vi "Run.vi"(7 "Tester":refnum<class "Tester.lvclass">, 8 "error in (no error)":errorcluster, 11 "Step in":refnum<class "Step.lvclass">) -> (0 "error out":errorcluster, 3 "Step out":refnum<class "Step.lvclass">)   [LabVIEW 2020, in "Tester.lvlib" / "Step.lvclass"]
uses:
  Step.lvclass
  Tester/Tester.lvclass
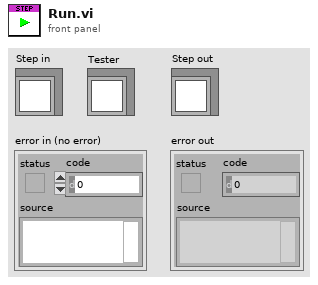
[diagram p1: front panel]
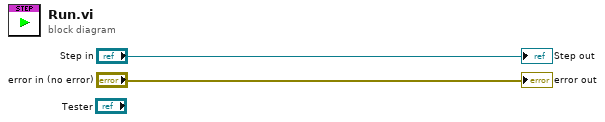
[diagram p0: block diagram]
diagram:
  "error out" <- "error in (no error)"
  "Step out" <- "Step in"
